vi "GUI_Target.vi"() -> ()   [LabVIEW 2013]
uses:
  shared programs/GUI_Template/GUI_master/tcp_new_data_event.ctl
  shared programs/GUI_Template/GUI_master/tcp new data cluster.ctl
  <vilib>/vision/Image Controls.llb/IMAQ Image.ctl
panel:
  in  "OD1":u16(ring)
  in  "OD2":u16(ring)
  in  "OD3":u16(ring)
  in  "OD4":u16(ring)
  in  "roi::5":bool caption="Blank Button"
  in  "trigger::5":bool caption="Blank Button"
  in  "exposure::5":dbl=0.001 caption="Exposure" min=3.8e-05 max=1.0 format="%_4p"
  in  "centroidx::5":dbl=0.001 caption="X" min=0.0 max=0.0
  in  "centroidy::5":dbl=0.001 caption="Y" min=0.0 max=0.0
  out "Display5":T1(plugin-control) caption="M1 Cam"
  in  "Target.X::5":dbl=0.001 caption="X" min=0.0 max=2000.0
  in  "Target.Y::5":dbl=0.001 caption="Y" min=0.0 max=2000.0
  in  "size5":dbl=25.0 caption="Size" min=0.0 max=0.0
  out "image::5":T1(plugin-control) caption="M1 Cam"
  in  "GUIdevice 5":string="HPD_CCD"
  in  "stepsize::3":dbl caption="Step Size" min=0.0 max=1.0
  in  "stepsize::4":dbl caption="Step Size" min=0.0 max=1.0
  in  "relativeMove.Axis 1neg::4":bool caption="Right"
  in  "relativeMove.Axis 1pos::4":bool caption="Left"
  in  "relativeMove.Axis 2pos::4":bool caption="Down"
  in  "relativeMove.Axis 2neg::4":bool caption="relativemove.Axis 3neg::6"
  in  "relativeMove.Axis 1neg::3":bool
  in  "relativeMove.Axis 1pos::3":bool
  in  "relativeMove.Axis 2pos::3":bool
  in  "relativeMove.Axis 2neg::3":bool
  in  "GUIdevice 4":string="HPD_ESP2"
  in  "GUIdevice 3":string="HPD_ESP1"
  out "image::2":T1(plugin-control) caption="M1 Cam"
  in  "stop":bool
  in  "LP":u16(ring)
  out "error IO 2":errorcluster
  out "tcp data event":T2
  in  "GUIdevice 1":string="SmaractFilter-1"
  in  "Position.Channel 3::1":dbl caption="Position (LP Mode)" min=2.0 max=60.0 format="%#_6p"
  in  "Position.Channel 5::1":dbl caption="Position OD4 (CH5)" min=2.0 max=50.0 format="%#_6p"
  in  "Position.Channel 4::1":dbl caption="Position OD2 (CH4)" min=2.0 max=50.0 format="%#_6p"
  in  "Position.Channel 2::1":dbl caption="Position OD3 (CH2)" min=2.0 max=52.0 format="%#_6p"
  in  "Position.Channel 1::1":dbl caption="Position OD1 (CH1)" min=2.0 max=50.0 format="%#_6p"
  in  "filter.Channel 5::1":enum16{"off", "on"}(ring) caption="OD4 (CH5)"
  in  "filter.Channel 4::1":enum16{"off", "on"}(ring) caption="OD2 (CH4)"
  in  "filter.Channel 2::1":enum16{"off", "on"}(ring) caption="OD3 (CH2)"
  in  "filter.Channel 1::1":enum16{"off", "on"}(ring) caption="OD1 (CH1)"
  in  "roi::2":bool caption="Blank Button"
  in  "size2":dbl=20.0 caption="Size" min=0.0 max=0.0
  in  "Target.X::2":dbl=0.001 caption="X" min=0.0 max=2000.0
  in  "Target.Y::2":dbl=0.001 caption="Y" min=0.0 max=2000.0
  in  "centroidx::2":dbl=0.001 caption="X" min=0.0 max=0.0
  in  "centroidy::2":dbl=0.001 caption="Y" min=0.0 max=0.0
  in  "trigger::2":bool caption="Blank Button"
  in  "exposure::2":dbl=0.001 caption="Exposure" min=3.8e-05 max=1.0 format="%_4p"
  in  "GUIdevice 2":string="Bella_LP_Mode"
  out "Display2":T1(plugin-control) caption="M1 Cam"
  # "BELLA TARGET AREA MAP"
  # "Centroid"
  # "Target"
  # "HPD_ESP1"
  # "HPD_ESP2"
  # "Centroid"
  # "Target"
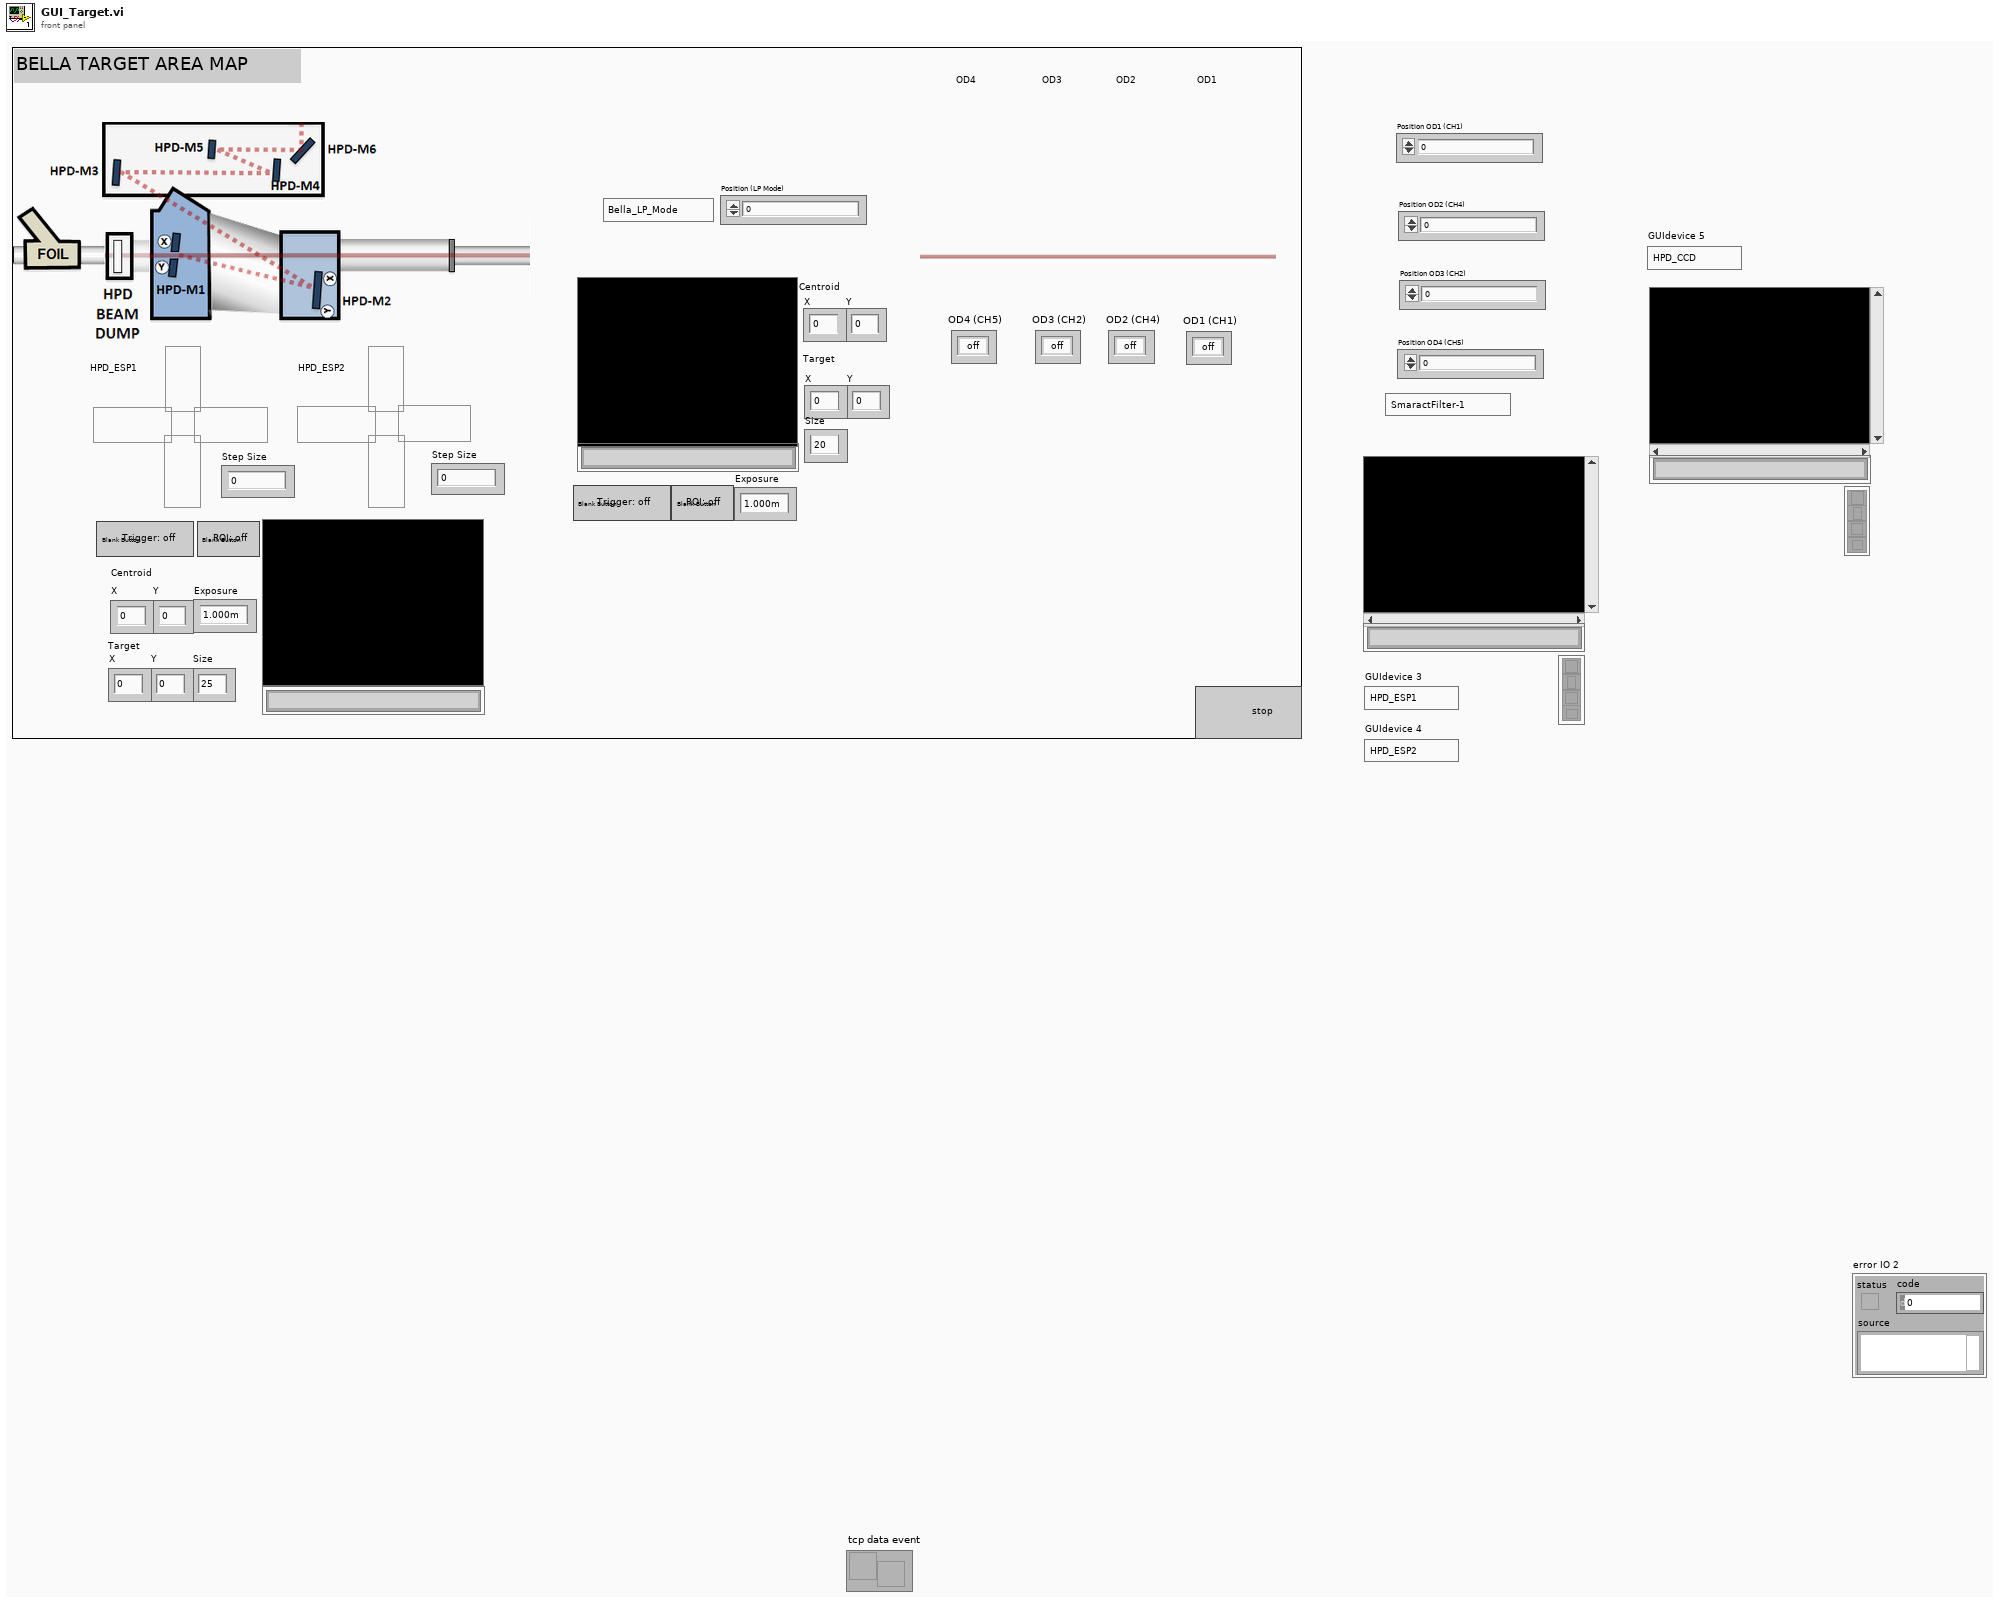
[diagram p1: front panel]
types:
  T1 = typedef "IMAQ Image.ctl" = refnum<image>
  T2 = typedef "tcp_new_data_event.ctl" = refnum<user-event>
  T3 = typedef "Image Type" = u32
  T4 = cluster{"Last update M1":u32, "Last update M2":u32, "Last update M4":u32, "Last update M5":u32, "Last update LPD":u32}
  T5 = typedef "tcp new data cluster.ctl" = cluster{"EventEnum":enum16{"new data", "connection status update"}, "Device name":string}
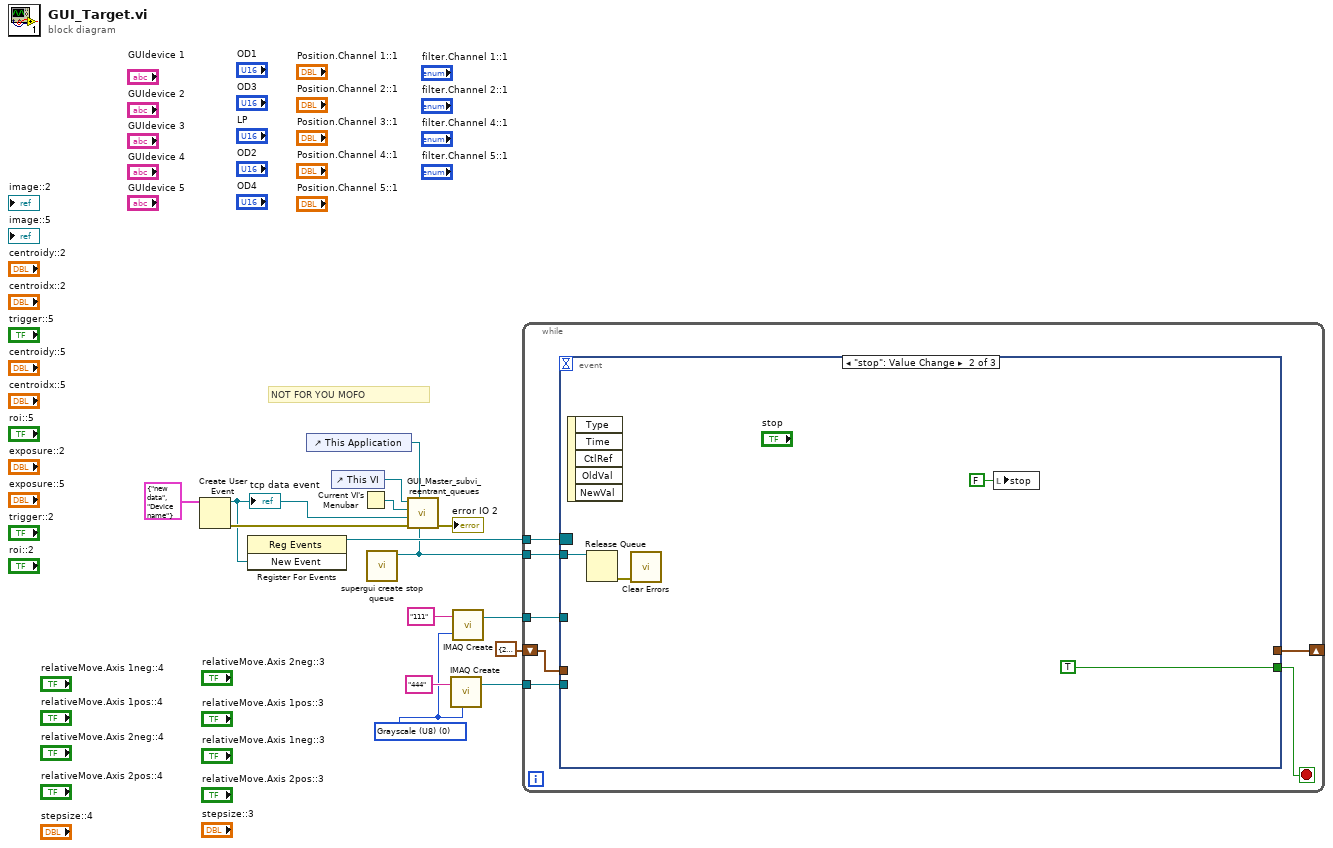
[diagram p0: block diagram]
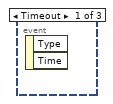
[diagram p2: hidden frame]
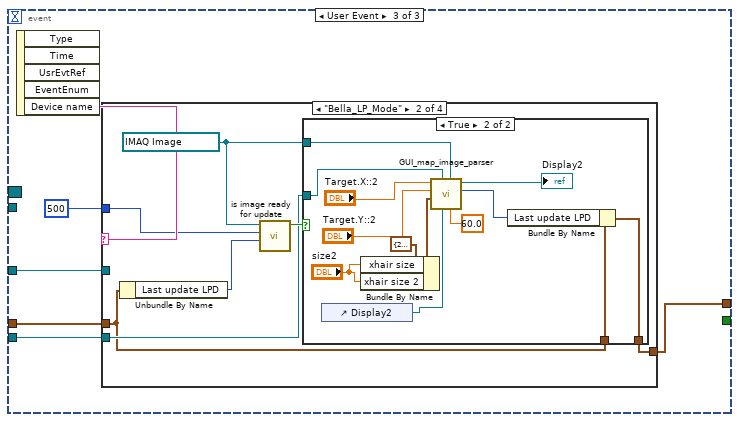
[diagram p3: hidden frame]
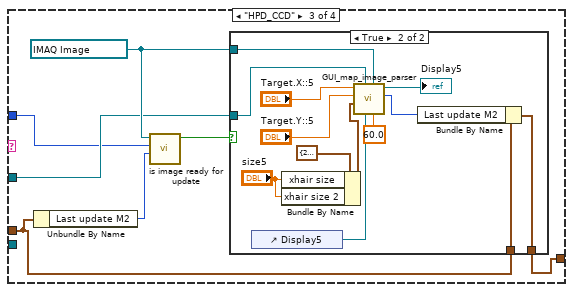
[diagram p6: hidden frame]
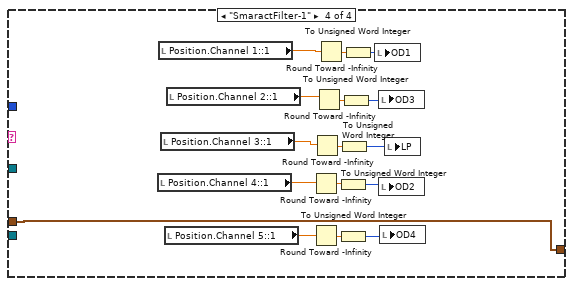
[diagram p8: hidden frame]
diagram:
  w3 = T3 0 items=["Grayscale (U8)", "Grayscale (I16)", "Grayscale (SGL)", "Complex (CSG)", "RGB (U32)", "HSL (U32)", "RGB (U64)", "Grayscale (U16)"] ("Image Type")
  # "NOT FOR YOU MOFO"
  n1 = Create User Event(user event datatype=T5 {"EventEnum"=enum."new data", "Device name"="Device name"} ("New Event")) -> (user event=w10:refnum<user-event>, error out=w11:errorcluster)  [unwired: 1 in]
  "tcp data event" <- w10
  n2 = register-events(w10) -> (reference out=w8:refnum<event-registration>)  [unwired: 2 in, 1 out]
  n3 = control-ref of="This Application"() -> (w9:refnum<vi>)
  n4 = control-ref of="This VI"() -> (w14:refnum<vi>)
  n5 = Current VI's Menubar() -> (w13:refnum<k9>)
  n6 = call "supergui create stop queue.vi"() -> ("STOP Queue out"=w1:refnum<queue>)  [unwired: 11 in]
  n7 = call "GUI_Master_subvi_reentrant_queues.vi"("STOP Queue in"=w1, "This Application"=w9, "error in (no error)"=w11, "tcp data event"=w10, "Caller menu reference"=w13, "Caller VI ref"=w14) -> ("error out"=→"error IO 2":errorcluster)  [unwired: 5 in]
  n8 = call "IMAQ Create"("Image Name"="444", "Image Type"=w3) -> ("New Image"=w5:T1)  [unwired: 3 in, 1 out]
  n9 = call "IMAQ Create"("Image Name"="111", "Image Type"=w3) -> ("New Image"=w2:T1)  [unwired: 3 in, 1 out]
  n10 = while {
    tunnel: w8 -> [w21]
    shift-right: [w18] -> _
    shift-left: T4 {"Last update M1"=200, "Last update M2"=200, "Last update M4"=200, "Last update M5"=200, "Last update LPD"=200} -> [w19]
    tunnel: w5 -> [w20]
    tunnel: w2 -> [w17]
    tunnel: w1 -> [w16]
    stop <- w22 stop-if-true
    n11 = event shown="[1] \"stop\": Value Change" {
      selector: w21 -> [_ _ _]
      dyn-events: _ -> [_ _ _]
      timeout: _ -> [_ _ _]
      tunnel: [_ TRUE _] -> w22
      tunnel: w20 -> [_ _ w31]
      tunnel: w19 -> [_ _ w29]
      tunnel: [_ _ w28] -> w18
      tunnel: w17 -> [_ _ w27]
      tunnel: w16 -> [_ w24 _]
      event Timeout {
        n12 = event-data() -> ()  [unwired: 1 in, 2 out]
      }
      event "stop": Value Change {
        n13 = event-data() -> ()  [unwired: 1 in, 5 out]
        n14 = Release Queue(queue=w24) -> (error out=w23:errorcluster)  [unwired: 2 in, 2 out]
        n15 = call <vilib>:"Clear Errors.vi"("error in (no error)"=w23) -> ()  [unwired: 6 in, 1 out]
        n16 = local write "stop"(FALSE ("stop")) -> ()
      }
      event User Event {
        n17 = event-data() -> ("Device name"=w32:string)  [unwired: 1 in, 4 out]
        n18 = case shown="\"Bella_LP_Mode\"" w32 {
          tunnel: w31 -> [_ w36 _ _]
          tunnel: u32 500 ("x-y") -> [_ w37 w55 _]
          tunnel: w29 -> [w33 w35 w57 w76]
          tunnel: [w33 w34 w58 w76] -> w28
          tunnel: w27 -> [_ _ w56 _]
          frame Default {
          }
          frame "Bella_LP_Mode" {
            w38 = T1 refnum ("New Image")
            n19 = Unbundle By Name(w35) -> ("Last update LPD"=w39:u32)
            n20 = call "is image ready for update.vi"("Last update"=w39, "min time between updates"=w37, "image ref in"=w38) -> ("update image"=w40:bool)  [unwired: 8 in]
            n21 = case shown="True" w40 {
              tunnel: w36 -> [_ w51]
              tunnel: w35 -> [w41 w54]
              tunnel: [w41 w53] -> w34
              tunnel: w38 -> [_ w52]
              frame False {
              }
              frame True {
                n22 = control-ref of="Display2"() -> (w47:refnum<vi>)
                n23 = Bundle By Name(cluster=cluster{"xhair size":dbl, "xhair size 2":dbl} {"xhair size"=20.0, "xhair size 2"=20.0} ("size"), "xhair size"="size2", "xhair size 2"="size2") -> (w42:cluster{"xhair size":dbl, "xhair size 2":dbl})
                n24 = call "GUI_map_image_parser.vi"("zoom#"=60.0, "Image Src"=w52, "Ctl Refnum"=w47, "Image Dst"=w51, "size"=w42, "target y"="Target.Y::2", "target x"="Target.X::2") -> ("ms timer out"=w49:u32, "Img out"=→"Display2":T1)  [unwired: 3 in]
                n25 = Bundle By Name(cluster=w54, "Last update LPD"=w49) -> (w53:T4)
              }
            }
          }
          frame "HPD_CCD" {
            w61 = T1 refnum ("New Image")
            n26 = Unbundle By Name(w57) -> ("Last update M2"=w59:u32)
            n27 = call "is image ready for update.vi"("Last update"=w59, "min time between updates"=w55, "image ref in"=w61) -> ("update image"=w60:bool)  [unwired: 8 in]
            n28 = case shown="True" w60 {
              tunnel: w56 -> [_ w72]
              tunnel: w57 -> [w62 w75]
              tunnel: [w62 w74] -> w58
              tunnel: w61 -> [_ w73]
              frame False {
              }
              frame True {
                n29 = control-ref of="Display5"() -> (w69:refnum<vi>)
                n30 = Bundle By Name(cluster=cluster{"xhair size":dbl, "xhair size 2":dbl} {"xhair size"=20.0, "xhair size 2"=20.0} ("size"), "xhair size"="size5", "xhair size 2"="size5") -> (w63:cluster{"xhair size":dbl, "xhair size 2":dbl})
                n31 = call "GUI_map_image_parser.vi"("zoom#"=60.0, "Image Src"=w73, "Ctl Refnum"=w69, "Image Dst"=w72, "size"=w63, "target y"="Target.Y::5", "target x"="Target.X::5") -> ("ms timer out"=w67:u32, "Img out"=→"Display5":T1)  [unwired: 3 in]
                n32 = Bundle By Name(cluster=w75, "Last update M2"=w67) -> (w74:T4)
              }
            }
          }
          frame "SmaractFilter-1" {
            n33 = local read "Position.Channel 4::1"() -> (w78:dbl)
            n34 = local read "Position.Channel 1::1"() -> (w81:dbl)
            n35 = local read "Position.Channel 3::1"() -> (w79:dbl)
            n36 = local read "Position.Channel 5::1"() -> (w77:dbl)
            n37 = local read "Position.Channel 2::1"() -> (w80:dbl)
            n38 = Round Toward -Infinity(1:w78) -> (0:w90:dbl)
            n39 = Round Toward -Infinity(1:w77) -> (0:w87:dbl)
            n40 = Round Toward -Infinity(1:w79) -> (0:w89:dbl)
            n41 = Round Toward -Infinity(1:w80) -> (0:w84:dbl)
            n42 = Round Toward -Infinity(1:w81) -> (0:w82:dbl)
            n43 = To Unsigned Word Integer(number=w90) -> (unsigned 16bit integer=w85:u16)
            n44 = To Unsigned Word Integer(number=w87) -> (unsigned 16bit integer=w88:u16)
            n45 = To Unsigned Word Integer(number=w89) -> (unsigned 16bit integer=w91:u16)
            n46 = To Unsigned Word Integer(number=w84) -> (unsigned 16bit integer=w86:u16)
            n47 = To Unsigned Word Integer(number=w82) -> (unsigned 16bit integer=w83:u16)
            n48 = local write "OD1"(w83) -> ()
            n49 = local write "OD3"(w86) -> ()
            n50 = local write "OD2"(w85) -> ()
            n51 = local write "OD4"(w88) -> ()
            n52 = local write "LP"(w91) -> ()
          }
        }
      }
    }
  }
